vi "UDP Receive.vi"(8 "error in (no error)":errorcluster, 9 "Transfer Group Rx parameters":T1={"Transfers Rx"=[], "max size"=548} {"max size" format="%d bytes"; "Transfers Rx"."source address" format="%d ms"; "Transfers Rx"."timeout" format="%d bytes"}, 10 "Transfer Group":refnum<class "Transfer Group.lvclass">, 11 "UDP Transceiver in":refnum<class "UDP Transceiver.lvclass">) -> (0 "error out":errorcluster, 3 "UDP Transceiver out":refnum<class "UDP Transceiver.lvclass">)   [LabVIEW 2017, in "UDP Transceiver.lvlib" / "UDP Transceiver.lvclass"]
uses:
  UDP Transceiver.lvclass
  UDP Transfer Group Receive Parameters.ctl
  UDP Transfer Receive Parameters.ctl
  Builds/Data Sharing Framework/Current/Data Sharing Framework Core/DSF Core.lvlibp/Engine/Classes/Transfer/Transfer Group.lvclass
  Builds/Data Sharing Framework/Current/Data Sharing Framework Core/DSF Core.lvlibp/Engine/Classes/Transfer/Transfer Group.lvclass/Transfer Group.ctl
  Builds/Data Sharing Framework/Current/Data Sharing Framework Core/DSF Core.lvlibp/Engine/Classes/Transfer/Transfer.lvclass/Transfer.ctl
  Builds/Data Sharing Framework/Current/Data Sharing Framework Core/DSF Core.lvlibp/Engine/Classes/Buffer/Buffer.lvclass/Buffer.ctl
  Builds/Data Sharing Framework/Current/Data Sharing Framework Core/DSF Core.lvlibp/Engine/Classes/Transfer/Transfer.Get String Buffer.vi
  Builds/Data Sharing Framework/Current/Data Sharing Framework Core/DSF Core.lvlibp/Engine/Classes/Buffer/Buffer.Get Buffer Size.vi
  Builds/Data Sharing Framework/Current/Data Sharing Framework Core/DSF Core.lvlibp/Engine/Classes/Buffer/Buffer.Write.vi
  Builds/Data Sharing Framework/Current/Data Sharing Framework Core/DSF Core.lvlibp/Engine/Classes/Buffer/Buffer.Write.1D.U8.vi
  UDP Errors.vi
  UDP Size Mismatch Error.vi
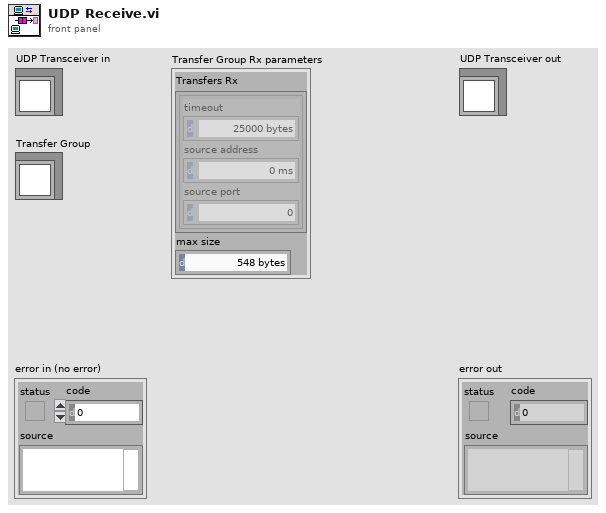
[diagram p1: front panel]
types:
  T1 = typedef "UDP Transceiver.lvlib/UDP Transceiver.lvclass/UDP Transfer Group Receive Parameters.ctl" = cluster{"Transfers Rx":T2[], "max size":i32}
  T2 = typedef "UDP Transceiver.lvlib/UDP Transceiver.lvclass/UDP Transfer Receive Parameters.ctl" = cluster{"timeout":i32, "source address":u32, "source port":u16}
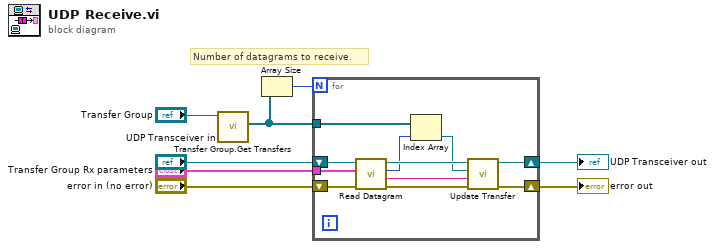
[diagram p0: block diagram]
diagram:
  # "Number of datagrams to receive."
  n1 = call "Transfer Group.Get Transfers.vi"("Transfer Group in"="Transfer Group") -> ("Transfers"=w3:refnum<class "Transfer.lvclass">[])  [unwired: 9 in, 1 out]
  n2 = Array Size(array=w3) -> (size(s)=w4:i32)
  n3 = for {
    N: w4 -> [_]
    shift-right: [w9] -> w6
    shift-left: "error in (no error)" -> [w18]
    tunnel: w3 -> [w16]
    tunnel: "Transfer Group Rx parameters" -> [w17]
    shift-right: [w10] -> w1
    shift-left: "UDP Transceiver in" -> [w19]
    n4 = call "Read Datagram.vi"("error in (no error)"=w18, "Transfer Group Rx parameters"=w17, "UDP in"=w19) -> ("error out"=w14:errorcluster, "data"=w13:string, "Transfer index"=w11:i32, "UDP out"=w15:refnum<class "UDP Transceiver.lvclass">)  [unwired: 5 in]
    n5 = Index Array(array=w16, index=w11) -> (element=w12:refnum<class "Transfer.lvclass">)
    n6 = call "Update Transfer.vi"("error in (no error)"=w14, "data"=w13, "Transfer"=w12, "UDP Transceiver in"=w15) -> ("error out"=w9:errorcluster, "UDP Transceiver out"=w10:refnum<class "UDP Transceiver.lvclass">)  [unwired: 6 in]
  }
  "error out" <- w6
  "UDP Transceiver out" <- w1
